vi "U6 Multiple IO Example eAddGoGet.vi"() -> ()   [LabVIEW 2021]
panel:
  out "Read Values":T1 {"AIN3" format="%.6f"; "AIN2" format="%.6f"; "AIN1" format="%.6f"; "AIN0" format="%.6f"}
  in  "Write Values":T2 {"DAC1" format="%.4f"; "DAC0" format="%.4f"}
  out "Error Message":string
  in  "error in":errorcluster
  out "error out":errorcluster
  # "Outputs DAC0-DAC1 and FIO2-FIO3.  Aquires AIN0-AIN3 and FIO0-FIO1.  Uses USB on the first found U6.\n\nThis uses eAddGoGet from the UD driver, rather than the LabVIEW utility AddS-Go-Get.vi.  The utility\nVI has better/easier error handling and is normally preferred, but eAddGoGet is a single call to the UD driver\nso often preferred if you will have parallel driver calls to the same handle within the same thread (none of\nour examples do this)."
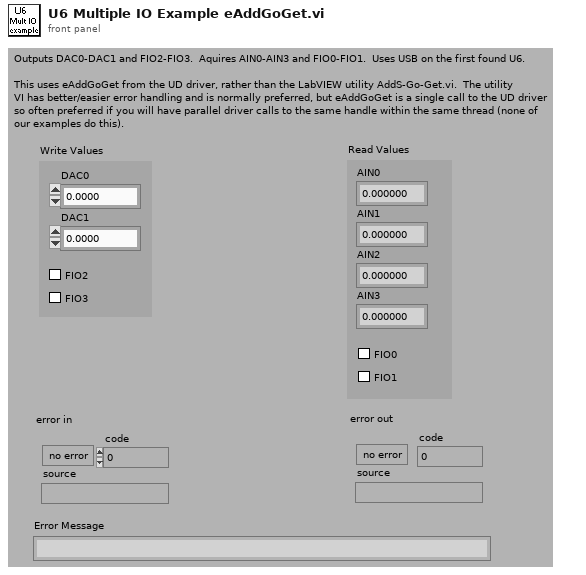
[diagram p1: front panel]
types:
  T1 = cluster{"AIN0":dbl, "AIN1":dbl, "AIN2":dbl, "AIN3":dbl, "FIO0":bool, "FIO1":bool}
  T2 = cluster{"DAC0":dbl, "DAC1":dbl, "FIO2":bool, "FIO3":bool}
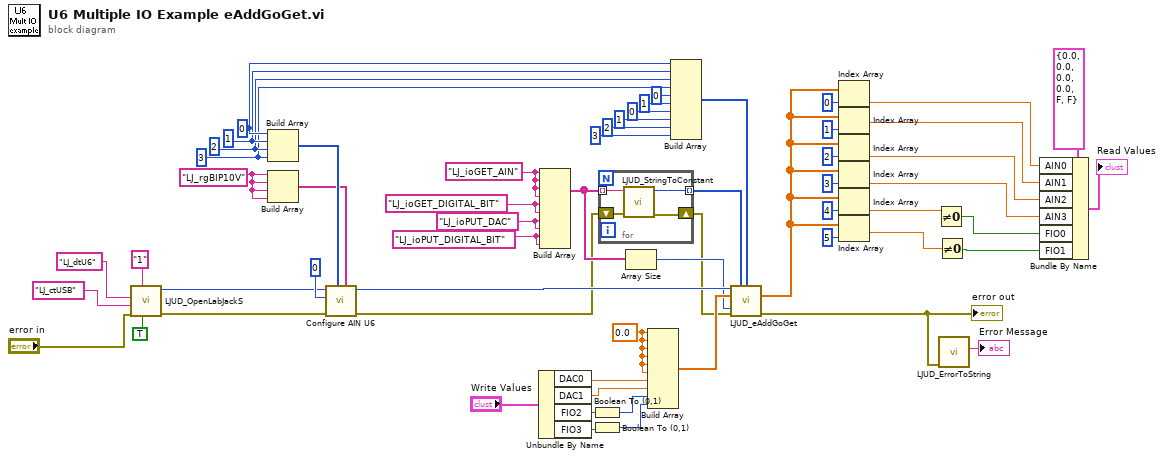
[diagram p0: block diagram]
diagram:
  w41 = 0.0 ("Input Element")
  w52 = "LJ_ioPUT_DIGITAL_BIT" ("IOType")
  w53 = "LJ_ioPUT_DAC" ("IOType")
  w55 = "LJ_ioGET_AIN" ("IOType")
  w48 = 3 ("SettlingFactor")
  w49 = 2 ("SettlingFactor")
  w50 = 1 ("SettlingFactor")
  w51 = 0 ("SettlingFactor")
  w26 = "LJ_rgBIP10V" ("AIN Range")
  w54 = "LJ_ioGET_DIGITAL_BIT" ("IOType")
  n1 = call "LJUD_OpenLabJackS.vi"("FirstFound"=TRUE, "Address"="1", "error in"="error in", "ConnectionType"="LJ_ctUSB", "DeviceType"="LJ_dtU6") -> ("error out"=w28:errorcluster, "Handle"=w24:i32)  [unwired: 4 in, 1 out]
  n2 = Build Array(w51, w50, w49, w48) -> (w27:i32[])
  n3 = Build Array(w26, w26, w26, w26) -> (w25:string[])
  n4 = call "Configure AIN U6.vi"("Ranges"=w25, "Positive Channels"=w27, "error in"=w28, "Resolution"=0, "Handle In"=w24) -> ("error out"=w2:errorcluster, "Handle Out"=w58:i32)  [unwired: 5 in]
  n5 = Unbundle By Name("Write Values") -> ("DAC0"=w36:dbl, "DAC1"=w35:dbl, "FIO2"=w34:bool, "FIO3"=w33:bool)
  n6 = Build Array(w55, w55, w55, w55, w54, w54, w53, w53, w52, w52) -> (w4:string[])
  n7 = Boolean To (0,1)(Boolean=w34) -> (0, 1=w40:i16)
  n8 = Boolean To (0,1)(Boolean=w33) -> (0, 1=w39:i16)
  n9 = for {
    shift-right: [w61] -> w1
    shift-left: w2 -> [w62]
    tunnel: w4 -> [w64] mode=indexing
    tunnel: [w63] -> w6 mode=indexing
    n10 = call "LJUD_StringToConstant.vi"("error in"=w62, "String"=w64) -> ("error out"=w61:errorcluster, "Constant Number"=w63:i32)  [unwired: 8 in]
  }
  n11 = Array Size(array=w4) -> (size(s)=w3:i32)
  n12 = Build Array(w41, w41, w41, w41, w41, w41, w36, w35, w40, w39) -> (w38:dbl[])
  n13 = Build Array(w51, w50, w49, w48, 0 ("Input Element"), 1 ("Input Element"), 0 ("Input Element"), 1 ("Input Element"), 2 ("Input Element"), 3 ("Input Element")) -> (w5:i32[])
  n14 = call "LJUD_eAddGoGet.vi"("Handle In"=w58, "aIOTypes"=w6, "aChannels"=w5, "Values Write"=w38, "NumRequests"=w3, "error in"=w1) -> ("Values Read"=w14:dbl[], "error out"=w57:errorcluster)  [unwired: 4 in, 4 out]
  "error out" <- w57
  n15 = Index Array(array=w14, index=0 ("Index")) -> (element=w12:dbl)
  n16 = Index Array(array=w14, index=1 ("Index")) -> (element=w11:dbl)
  n17 = Index Array(array=w14, index=2 ("Index")) -> (element=w10:dbl)
  n18 = Index Array(array=w14, index=3 ("Index")) -> (element=w9:dbl)
  n19 = Index Array(array=w14, index=4 ("Index")) -> (element=w8:dbl)
  n20 = Index Array(array=w14, index=5 ("Index")) -> (element=w7:dbl)
  n21 = Not Equal To 0?(x=w8) -> (x != 0?=w29:bool)
  n22 = Not Equal To 0?(x=w7) -> (x != 0?=w30:bool)
  n23 = call "LJUD_ErrorToString.vi"("error in"=w57) -> ("String"=→"Error Message":string)  [unwired: 10 in]
  n24 = Bundle By Name(cluster=T1 {"AIN0"=0.0, "AIN1"=0.0, "AIN2"=0.0, "AIN3"=0.0, "FIO0"=FALSE, "FIO1"=FALSE} ("Read Values"), "AIN0"=w12, "AIN1"=w11, "AIN2"=w10, "AIN3"=w9, "FIO0"=w29, "FIO1"=w30) -> (→"Read Values":T1)
